vi "LMT data analyse.vi"(11 "Datain":string) -> (3 "Dataout":string[](array[string]))   [LabVIEW 2017]
uses:
  <vilib>/regexp/Match Regular Expression.xnode
panel:
  out "为空？":bool
  out "数组":string[](array[string])
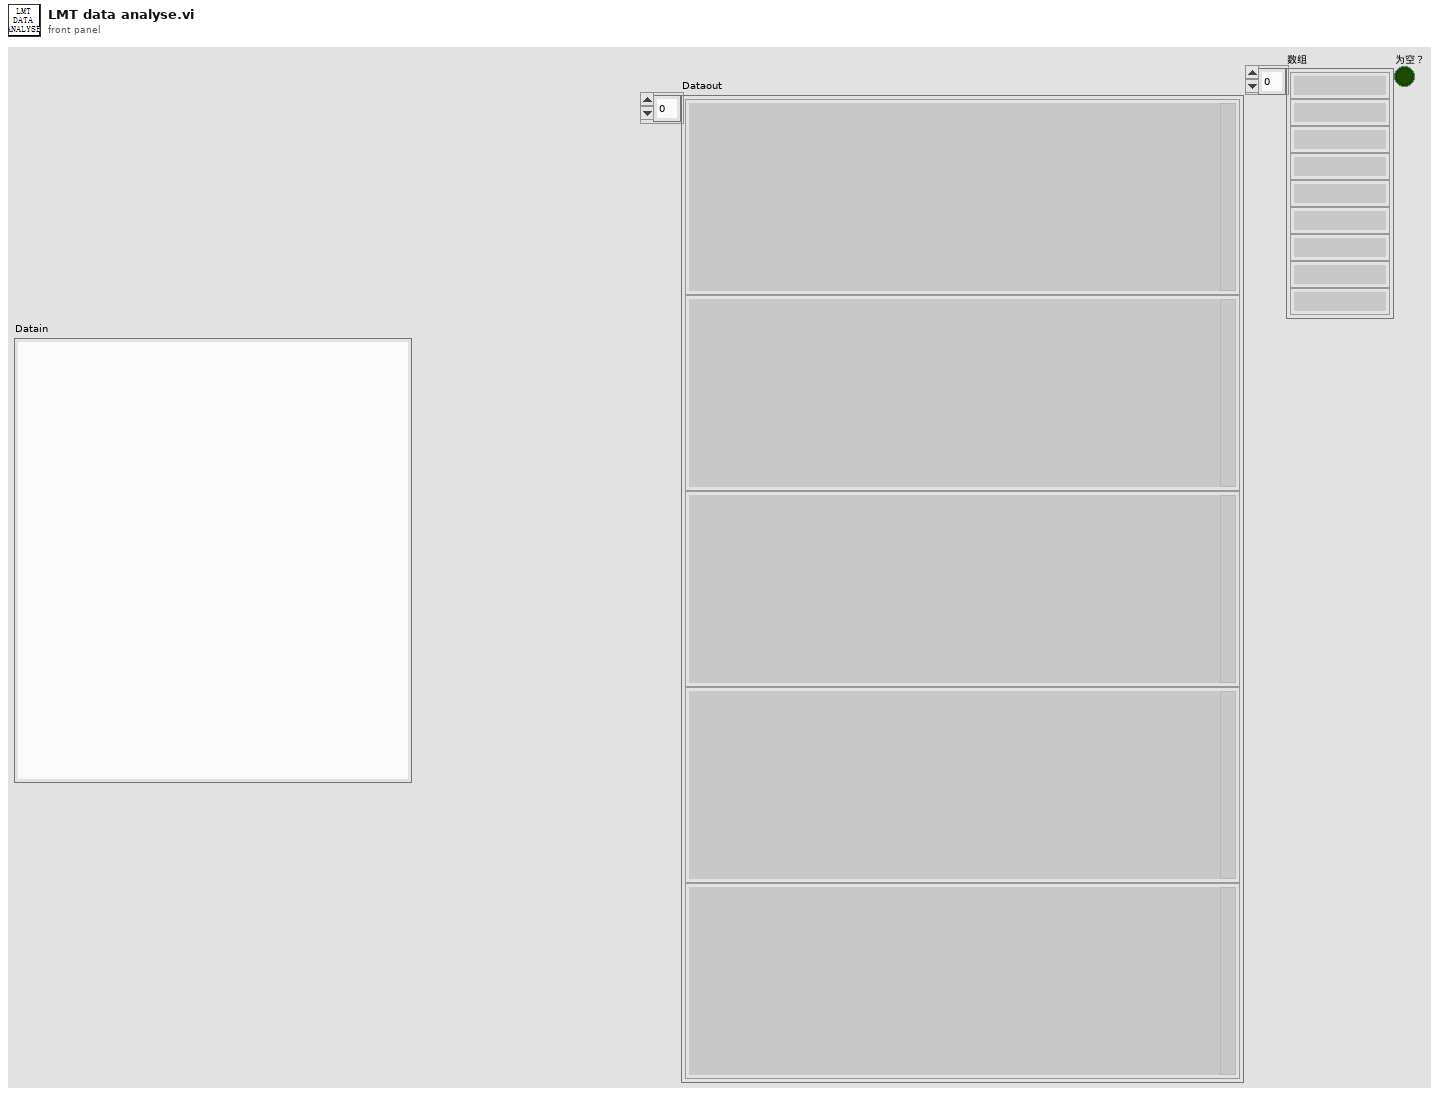
[diagram p1: front panel]
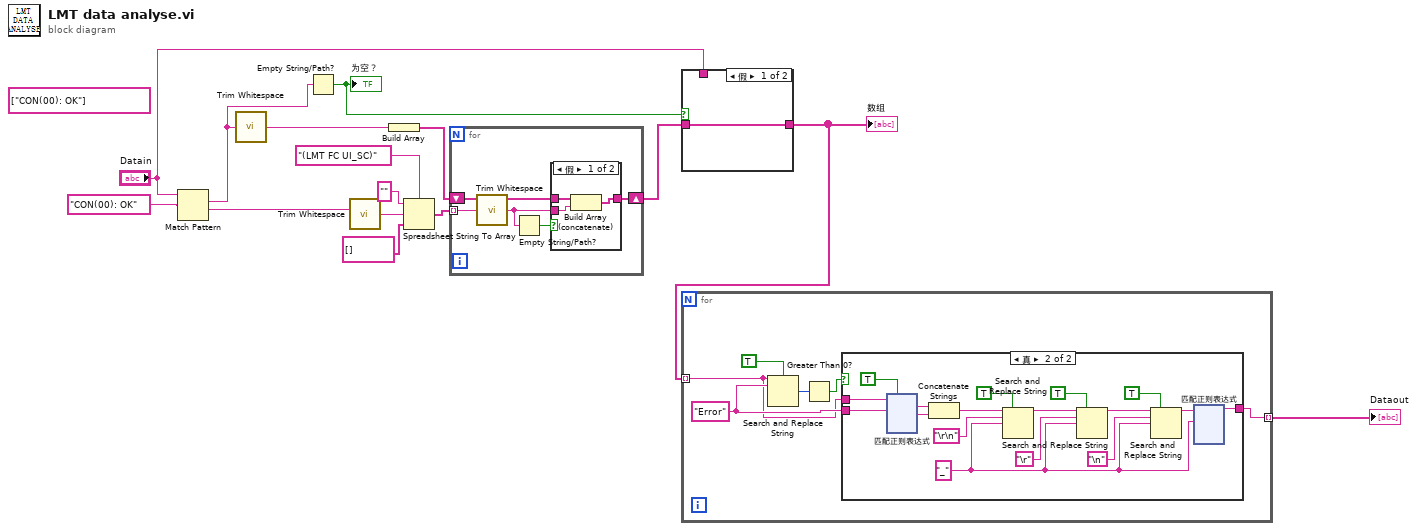
[diagram p0: block diagram]
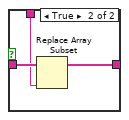
[diagram p2: hidden frame]
diagram:
  (unwired) string[] ["CON(00): OK"]
  n1 = Match Pattern(string="Datain", regular expression="CON(00): OK" ("正则表达式")) -> (match substring=w5:string, after substring=w12:string)  [unwired: 1 in, 2 out]
  n2 = call <vilib>:"Trim Whitespace.vi"("string"=w5) -> ("trimmed string"=w7:string)  [unwired: 1 in]
  n3 = Empty String/Path?(string/path=w5) -> (empty?=w3:bool)
  "为空？" <- w3
  n4 = call <vilib>:"Trim Whitespace.vi"("string"=w12) -> ("trimmed string"=w11:string)  [unwired: 1 in]
  n5 = Build Array(w7) -> (w9:string[])
  n6 = Spreadsheet String To Array(delimiter (Tab)="(LMT FC UI_SC)" ("搜索字符串"), format string="" ("格式字符串"), spreadsheet string=w11, array type (2D Dbl)=string[] []) -> (array=w10:string[])
  n7 = for {
    tunnel: w10 -> [w19] mode=indexing
    shift-right: [w18] -> w4
    shift-left: w9 -> [w17]
    n8 = call <vilib>:"Trim Whitespace.vi"("string"=w19) -> ("trimmed string"=w16:string)  [unwired: 1 in]
    n9 = Empty String/Path?(string/path=w16) -> (empty?=w20:bool)
    n10 = case shown="假" w20 {
      tunnel: w16 -> [w22 _]
      tunnel: [w23 w24] -> w18
      tunnel: w17 -> [w21 w24]
      frame False {
        n11 = Build Array (concatenate)(w21, w22) -> (w23:string[])
      }
      frame True {
      }
    }
  }
  n12 = case shown="假" w3 {
    tunnel: w4 -> [w25 w28]
    tunnel: "Datain" -> [_ w27]
    tunnel: [w25 w26] -> w1
    frame False {
    }
    frame True {
      n13 = Replace Array Subset(array=w28, new element=w27) -> (w26:string[])  [unwired: 1 in]
    }
  }
  "数组" <- w1
  n14 = for {
    tunnel: w1 -> [w30] mode=indexing
    tunnel: [w29] -> w6 mode=indexing
    w32 = "Error" ("搜索字符串")
    n15 = Search and Replace String(case sensitive?=TRUE ("忽略大小写？(F)"), input string=w30, search string=w32) -> (number of replacements=w33:i32)  [unwired: 5 in, 3 out]
    n16 = Greater Than 0?(x=w33) -> (x > 0?=w34:bool)
    n17 = case shown="真" w34 {
      tunnel: w30 -> [w35 w44]
      tunnel: w32 -> [_ w43]
      tunnel: [w35 w39] -> w29
      frame False {
      }
      frame True {
        w36 = "_"
        n18 = xnode "匹配正则表达式"("输入字符串"=w44, "正则表达式"=w43, "忽略大小写？(F)"=TRUE) -> ("所有匹配"=w40:string, "匹配之后"=w41:string)  [unwired: 3 in, 3 out]
        n19 = Concatenate Strings(w40, w41) -> (w38:string)
        n20 = Search and Replace String(replace all?=TRUE ("replace all? (F)"), input string=w38, search string="\r\n", replace string=w36) -> (result string=w52:string)  [unwired: 4 in, 3 out]
        n21 = Search and Replace String(replace all?=TRUE ("replace all? (F)"), input string=w52, search string="\r", replace string=w36) -> (result string=w45:string)  [unwired: 4 in, 3 out]
        n22 = Search and Replace String(replace all?=TRUE ("replace all? (F)"), input string=w45, search string="\n", replace string=w36) -> (result string=w37:string)  [unwired: 4 in, 3 out]
        n23 = xnode "匹配正则表达式"("输入字符串"=w37, "正则表达式"=w36) -> ("匹配之前"=w39:string)  [unwired: 4 in, 4 out]
      }
    }
  }
  "Dataout" <- w6
